vi "PublicElectricityNetwork.vi"(5 "Day of Year":u32, 6 "Unique Object Identifier":string, 7 "Day Time":u32, 8 "Error In":errorcluster, 10 "Energy flow IN":T5, 11 "DataFlowIN":T4) -> (0 "Error Out":errorcluster, 1 "Feeding into the \npublic grid":bool, 2 "Energy flow OUT":T5, 3 "DataFlowOUT":T4)   [LabVIEW 2017]
uses:
  classes/DataCollector.lvclass
  classes/DataHandler.lvclass
  classes/SimulationParameter.lvclass
panel:
  out "Simulation Parameter":T1
  in  "Operating Parameter":T2
  out "Control Parameter":T3
  out "List of Fieldelements":string[](array[string])
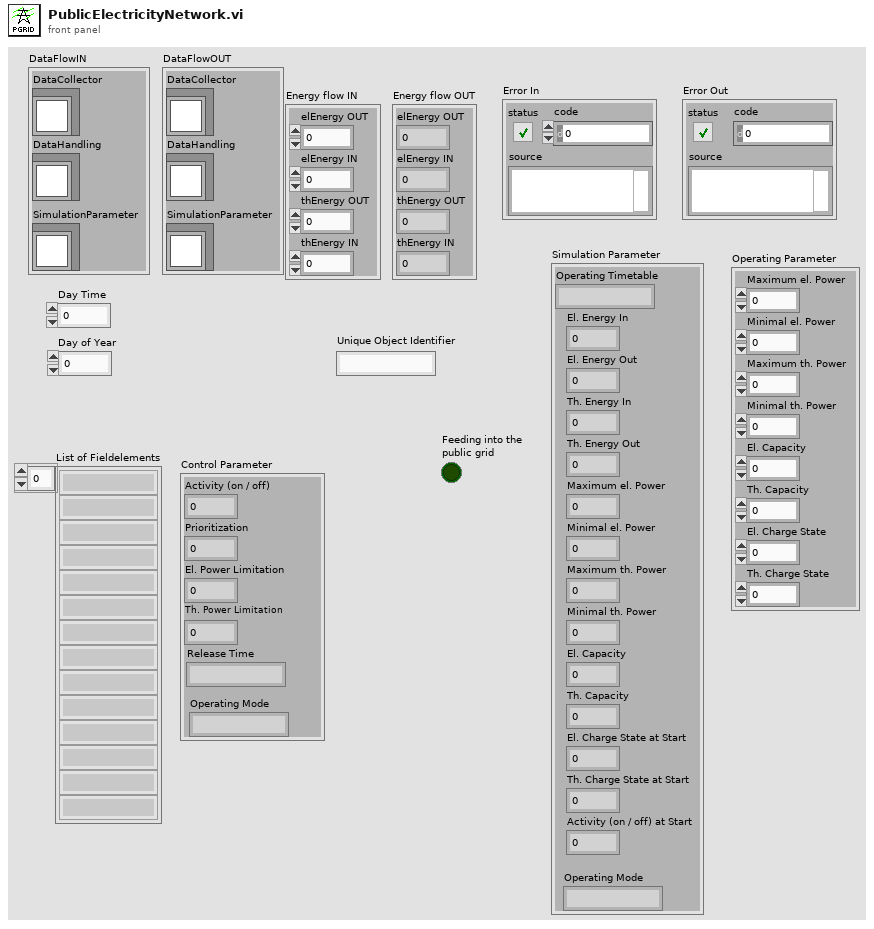
[diagram p1: front panel]
types:
  T1 = cluster{"Operating Timetable":string, "El. Energy In":dbl, "El. Energy Out":dbl, "Th. Energy In":dbl, "Th. Energy Out":dbl, "Maximum el. Power":dbl, "Minimal el. Power":dbl, "Maximum th. Power":dbl, "Minimal th. Power":dbl, "El. Capacity":dbl, "Th. Capacity":dbl, "El. Charge State at Start":dbl, "Th. Charge State at Start":dbl, "Activity (on / off) at Start":i64, "Operating Mode":string}
  T2 = cluster{"Maximum el. Power":dbl, "Minimal el. Power":dbl, "Maximum th. Power":dbl, "Minimal th. Power":dbl, "El. Capacity":dbl, "Th. Capacity":dbl, "El. Charge State":dbl, "Th. Charge State":dbl}
  T3 = cluster{"Activity (on / off)":i64, "Prioritization":i64, "El. Power Limitation":dbl, "Th. Power Limitation":dbl, "Release Time":string, "Operating Mode":string}
  T4 = cluster{"DataCollector":refnum<class "DataCollector.lvclass">, "DataHandling":refnum<class "DataHandler.lvclass">, "SimulationParameter":refnum<class "SimulationParameter.lvclass">}
  T5 = cluster{"elEnergy OUT":dbl, "elEnergy IN":dbl, "thEnergy OUT":dbl, "thEnergy IN":dbl}
  T6 = cluster{"elEnergy OUT":dbl, "thEnergy OUT":dbl, "thEnergy IN":dbl, "thEnergy IN":dbl}
  T7 = cluster{"Day Time":u32, "Day of Year":u32, cluster{"elEnergy OUT":dbl, "thEnergy OUT":dbl, "thEnergy IN":dbl, "thEnergy IN":dbl}, "Operating Parameter":cluster{"Maximum el. Power":dbl, "Minimal el. Power":dbl, "Maximum th. Power":dbl, "Minimal th. Power":dbl, "El. Capacity":dbl, "Th. Capacity":dbl, "El. Charge State":dbl, "Th. Charge State":dbl}, "Control Parameter":cluster{"Activity (on / off)":i64, "Prioritization":i64, "El. Power Limitation":dbl, "Th. Power Limitation":dbl, "Release Time":string, "Operating Mode":string}}
  T8 = cluster{"thEnergy IN":dbl, "thEnergy IN":dbl, "elEnergy OUT":dbl, "thEnergy OUT":dbl}
  T9 = cluster{"Day Time":u32, "Day of Year":u32, cluster{"thEnergy IN":dbl, "thEnergy IN":dbl, "elEnergy OUT":dbl, "thEnergy OUT":dbl}, "Operating Parameter":cluster{"Maximum el. Power":dbl, "Minimal el. Power":dbl, "Maximum th. Power":dbl, "Minimal th. Power":dbl, "El. Capacity":dbl, "Th. Capacity":dbl, "El. Charge State":dbl, "Th. Charge State":dbl}, "Control Parameter":cluster{"Activity (on / off)":i64, "Prioritization":i64, "El. Power Limitation":dbl, "Th. Power Limitation":dbl, "Release Time":string, "Operating Mode":string}}
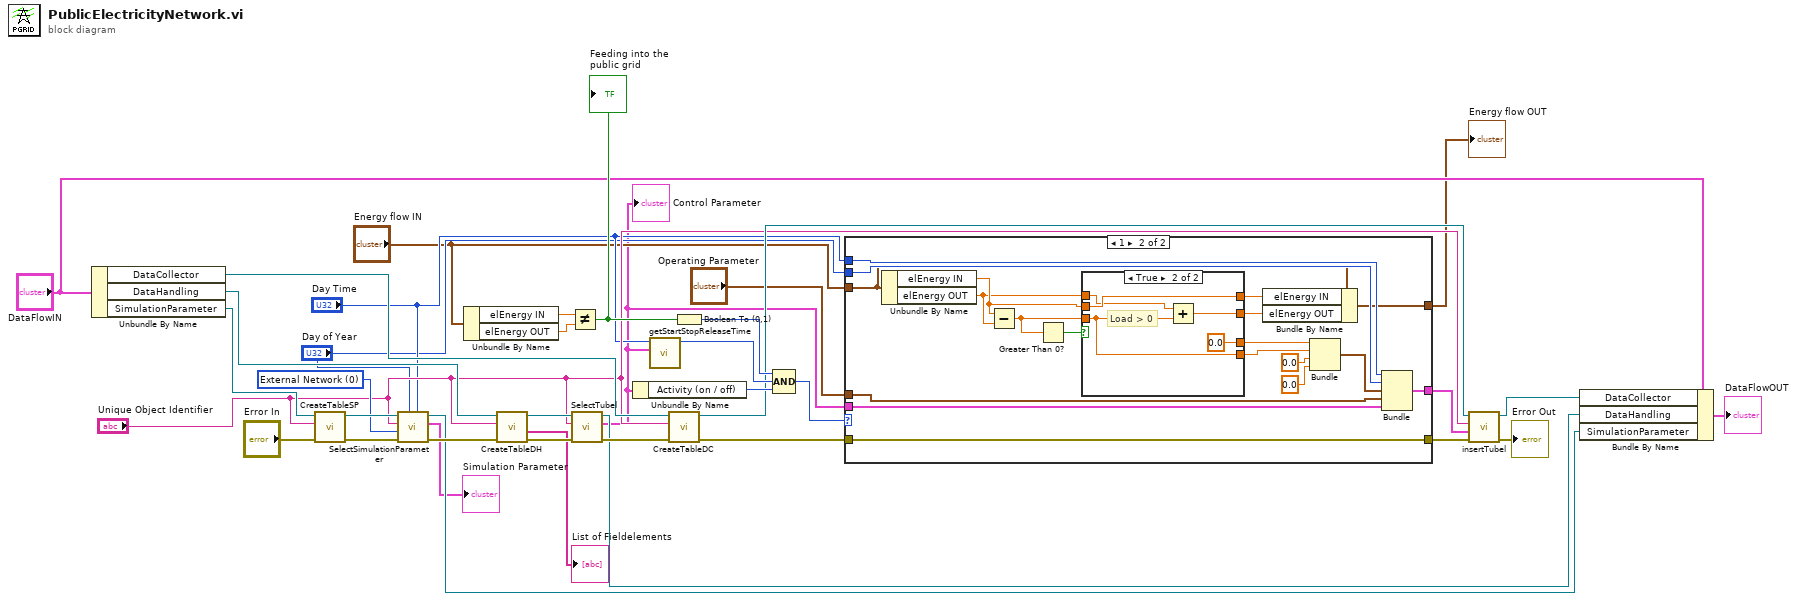
[diagram p0: block diagram]
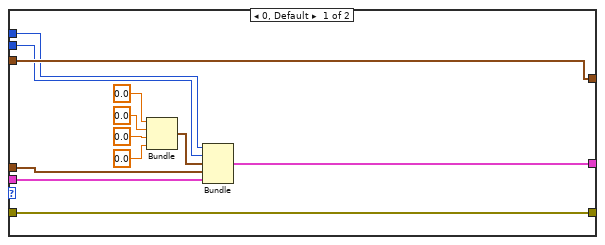
[diagram p2: hidden frame]
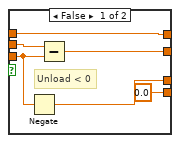
[diagram p3: hidden frame]
diagram:
  w16 = u16 0 items=["External Network", "Consumer", "Producer", "Sorage"] ("Type of Simulation")
  n1 = Unbundle By Name("DataFlowIN") -> ("DataCollector"=w37:refnum<class "DataCollector.lvclass">, "DataHandling"=w32:refnum<class "DataHandler.lvclass">, "SimulationParameter"=w27:refnum<class "SimulationParameter.lvclass">)
  n2 = call-dynamic "CreateTableSP.vi"("error in (no error)"="Error In", "Name of Table"="Unique Object Identifier", "SimulationParameter in"=w27) -> ("error out"=w30:errorcluster, "SimulationParameter out"=w29:refnum<class "SimulationParameter.lvclass">)  [unwired: 5 in, 2 out]
  n3 = call-dynamic "SelectSimulationParameter.vi"("Day of Year"="Day Time", "Day Time"="Day of Year", "error in (no error)"=w30, "Type of Simulation"=w16, "Unique Object Identifier"="Unique Object Identifier", "SimulationParameter in"=w29) -> ("error out"=w28:errorcluster, "Cluster"=→"Simulation Parameter":T1, "SimulationParameter out"=w26:refnum<class "SimulationParameter.lvclass">)  [unwired: 3 in]
  n4 = Unbundle By Name("Energy flow IN") -> ("elEnergy IN"=w19:dbl, "elEnergy OUT"=w18:dbl)
  n5 = call-dynamic "CreateTableDH.vi"("error in (no error)"=w28, "Name of Table"="Unique Object Identifier", "DataHandler in"=w32) -> ("error out"=w35:errorcluster, "List of Fieldelements"=→"List of Fieldelements":string[], "DataHandler out"=w33:refnum<class "DataHandler.lvclass">)  [unwired: 5 in, 1 out]
  n6 = Not Equal?(x=w19, y=w18) -> (x != y?=w17:bool)
  "Feeding into the \npublic grid" <- w17
  n7 = call-dynamic "SelectTubel.vi"("error in (no error)"=w35, "Unique Object Identifier"="Unique Object Identifier", "DataHandler in"=w33) -> ("error out"=w34:errorcluster, "Control Parameter"=w3:T3, "DataHandler out"=w31:refnum<class "DataHandler.lvclass">)  [unwired: 5 in, 1 out]
  "Control Parameter" <- w3
  n8 = Unbundle By Name(w3) -> ("Activity (on / off)"=w21:i64)
  n9 = call "getStartStopReleaseTime.vi"("Control Parameter"=w3, "Day Time"="Day Time") -> ("Activity (on / off)"=w22:i64)  [unwired: 9 in]
  n10 = call "CreateTableDC.vi"("error in (no error)"=w34, "Name of Table"="Unique Object Identifier", "DataCollector in"=w37) -> ("error out"=w14:errorcluster, "DataCollector out"=w15:refnum<class "DataCollector.lvclass">)  [unwired: 7 in]
  n11 = Boolean To (0,1)(Boolean=w17) -> (0, 1=w23:i16)
  n12 = Compound Arithmetic op=AND(w23, w22, w21) -> (w20:i64)
  n13 = case shown="1" w20 {
    tunnel: w14 -> [w48 w55]
    tunnel: [w48 w55] -> w25
    tunnel: "Day Time" -> [w41 w68]
    tunnel: "Day of Year" -> [w40 w67]
    tunnel: "Operating Parameter" -> [w43 w56]
    tunnel: "Energy flow IN" -> [w49 w66]
    tunnel: [w49 w65] -> w7
    tunnel: w3 -> [w38 w63]
    tunnel: [w39 w62] -> w24
    frame 0, Default {
      n14 = Bundle("elEnergy OUT"=0.0, "thEnergy OUT"=0.0, "thEnergy IN"=0.0, "thEnergy IN"=0.0) -> (w42:T6)  [unwired: 1 in]
      n15 = Bundle("Day Time"=w41, "Day of Year"=w40, w42, "Operating Parameter"=w43, "Control Parameter"=w38) -> (w39:T7)  [unwired: 1 in]
    }
    frame 1 {
      n16 = Unbundle By Name(w66) -> ("elEnergy IN"=w61:dbl, "elEnergy OUT"=w59:dbl)
      n17 = Subtract(x=w61, y=w59) -> (x-y=w60:dbl)
      n18 = Greater Than 0?(x=w60) -> (x > 0?=w54:bool)
      n19 = case shown="True" w54 {
        tunnel: w61 -> [w74 w79]
        tunnel: w60 -> [w70 w75]
        tunnel: w59 -> [w73 w78]
        tunnel: [w73 w79] -> w58
        tunnel: [w72 w76] -> w57
        tunnel: [w69 0.0 ("thEnergy IN")] -> w53
        tunnel: [0.0 ("thEnergy IN") w75] -> w52
        frame False {
          # "Unload < 0"
          n20 = Negate(x=w70) -> (-x=w69:dbl)
          n21 = Subtract(x=w74, y=w70) -> (x-y=w72:dbl)
        }
        frame True {
          # "Load > 0"
          n22 = Add(x=w78, y=w75) -> (x+y=w76:dbl)
        }
      }
      n23 = Bundle By Name(cluster=w66, "elEnergy IN"=w58, "elEnergy OUT"=w57) -> (w65:T5)
      n24 = Bundle("thEnergy IN"=w53, "thEnergy IN"=w52, "elEnergy OUT"=0.0, "thEnergy OUT"=0.0) -> (w64:T8)  [unwired: 1 in]
      n25 = Bundle("Day Time"=w68, "Day of Year"=w67, w64, "Operating Parameter"=w56, "Control Parameter"=w63) -> (w62:T9)  [unwired: 1 in]
    }
  }
  "Energy flow OUT" <- w7
  n26 = call-dynamic "insertTubel.vi"("error in (no error)"=w25, "Data Cluster"=w24, "Name of Table"="Unique Object Identifier", "DataCollector in"=w15) -> ("error out"=→"Error Out":errorcluster, "DataCollector out"=w36:refnum<class "DataCollector.lvclass">)  [unwired: 6 in]
  n27 = Bundle By Name(cluster="DataFlowIN", "DataCollector"=w36, "DataHandling"=w31, "SimulationParameter"=w26) -> (→"DataFlowOUT":T4)
